vi "Tuto_PWM.vi"() -> ()   [LabVIEW 2018]
uses:
  <vilib>/rvi/Emulation/niFpgaGetClockAttributes.vi
  <vilib>/rvi/Emulation/niFpgaSctlEmulationGetInTimedLoop.vi
  <vilib>/rvi/Emulation/niFpgaEmulationReportErrorSimple.vi
  <vilib>/rvi/eio/common/nirviEmuTemplateMethod_errors.vi
  <vilib>/rvi/Emulation/niFpgaCriticalErrorInLSC.vi
  <vilib>/eio/EIONode/EIONode.xnode
panel:
  in  "duty cycle (periods)":fxp<+,32,0>=0.06999999890103936 caption="Duty Cycle"
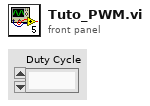
[diagram p1: front panel]
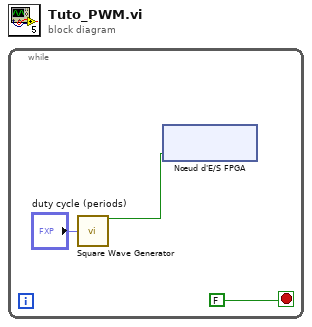
[diagram p0: block diagram]
diagram:
  n1 = while {
    stop <- FALSE stop-if-true
    n2 = call "Square Wave Generator"("duty cycle (periods)"="duty cycle (periods)") -> ("square wave out"=w3:bool)  [unwired: 14 in]
    n3 = xnode "Nœud d'E/S FPGA"("BB3_DIO0"=w3) -> ()  [unwired: 1 in, 1 out]
  }
